vi "ORS_sinc_interpol.vi"(8 "# zeros added":i32, 11 "In":dbl[](array[numeric])) -> (3 "Out":dbl[](array[numeric]))   [LabVIEW 2024]
uses:
  <vilib>/Analysis/2dsp.llb/Real FFT.vi
  <vilib>/Analysis/2dsp.llb/Inverse Real FFT.vi
  <vilib>/Analysis/NI_AALPro.lvlib
panel:
  out "In":dbl[](graph)
  out "Out":dbl[](graph)
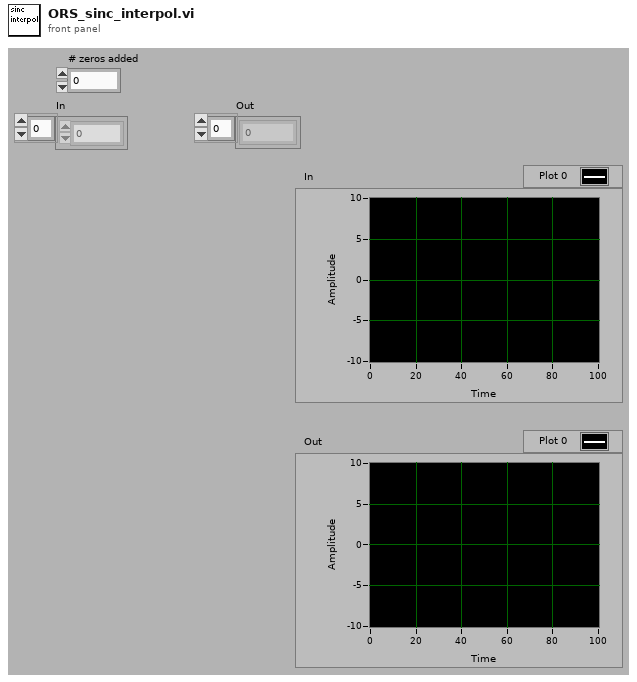
[diagram p1: front panel]
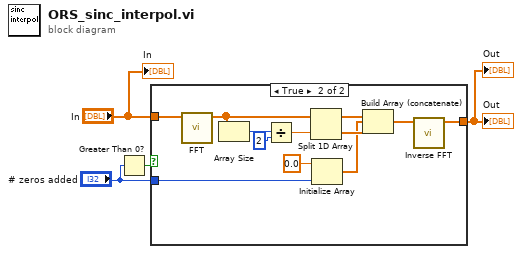
[diagram p0: block diagram]
diagram:
  n1 = Greater Than 0?(x="# zeros added") -> (x > 0?=w2:bool)
  n2 = case shown="True" w2 {
    tunnel: "# zeros added" -> [_ w17]
    tunnel: "In" -> [w5 w11]
    tunnel: [w5 w10] -> w3
    frame False {
    }
    frame True {
      n3 = call-poly <vilib>:"FFT.vi"("X"=w11) -> ("FFT {X}"=w9:cdb[])  [unwired: 9 in, 1 out]
      n4 = Array Size(array=w9) -> (size(s)=w8:i32)
      n5 = Divide(x=w8, y=2) -> (x/y=w7:dbl)
      n6 = Split 1D Array(array=w9, index=w7) -> (first subarray=w16:cdb[], second subarray=w15:cdb[])
      n7 = Initialize Array(0.0 ("element"), w17) -> (w12:dbl[])
      n8 = Build Array (concatenate)(w16, w12, w15) -> (w14:cdb[])
      n9 = call-poly <vilib>:"Inverse FFT.vi"("FFT {X}"=w14) -> ("X"=w10:dbl[])  [unwired: 9 in, 1 out]
    }
  }
  "Out" <- w3
  "Out" <- w3
  "In" <- "In"
